vi "Config Measure Event.vi"(0 "VISA resource name":refnum<visa-resource-name>, 1 "Configure Measurement (Disable)":enum8{"DISABLE", "ENABLE", "ASYNC"}(ring), 2 "Buffer 1":string, 3 "Buffer 2":string, 5 "Node In":string, 7 "Channel (Channel A)":T1, 9 "Function (Current)":T2(ring), 11 "error in":errorcluster, 12 "Measure Input Event":string="0") -> (4 "VISA resource name out":refnum<visa-resource-name>, 6 "Node Out":string, 14 "Command String":string, 15 "error out":errorcluster)   [LabVIEW 2009, in "Keithley 2600 Series.lvlib"]
doc: "This VI configures measurements for a subsequent sweep.\n\n<b>Functions and Attributes Used</b>\nsmuX.trigger.measure.action\nsmuX.trigger.measure.i( )\nsmuX.trigger.measure.v( )\nsmuX.trigger.measure.iv( )\nsmuX.trigger.measure.p( )\nsmuX.trigger.measure.r( )"
uses:
  <instrlib>/Keithley 2600 Series/Keithley 2600 Series.lvlib
  <instrlib>/Keithley 2600 Series/Public/Channel.ctl
  <instrlib>/Keithley 2600 Series/Private/GlobalVariables.vi
panel:
  # "(c) 2008 Keithley Instruments, Inc.  ALL RIGHTS RESERVED."
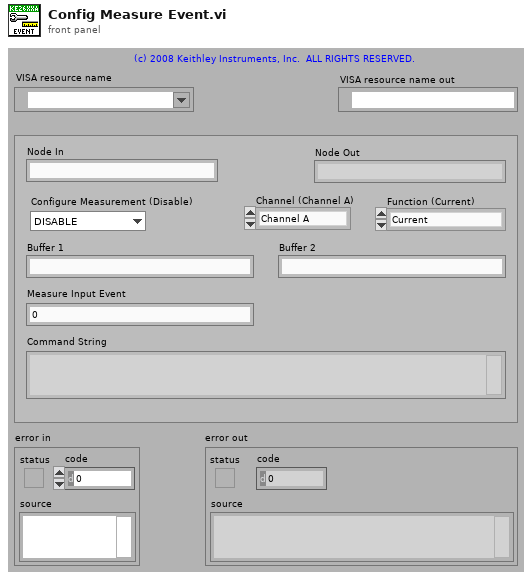
[diagram p1: front panel]
types:
  T1 = typedef "Keithley 2600 Series.lvlib/Channel.ctl" = enum32{"Channel A", "Channel B"}
  T2 = enum16{"Current", "Voltage", "IV", "Resistance", "Power"}
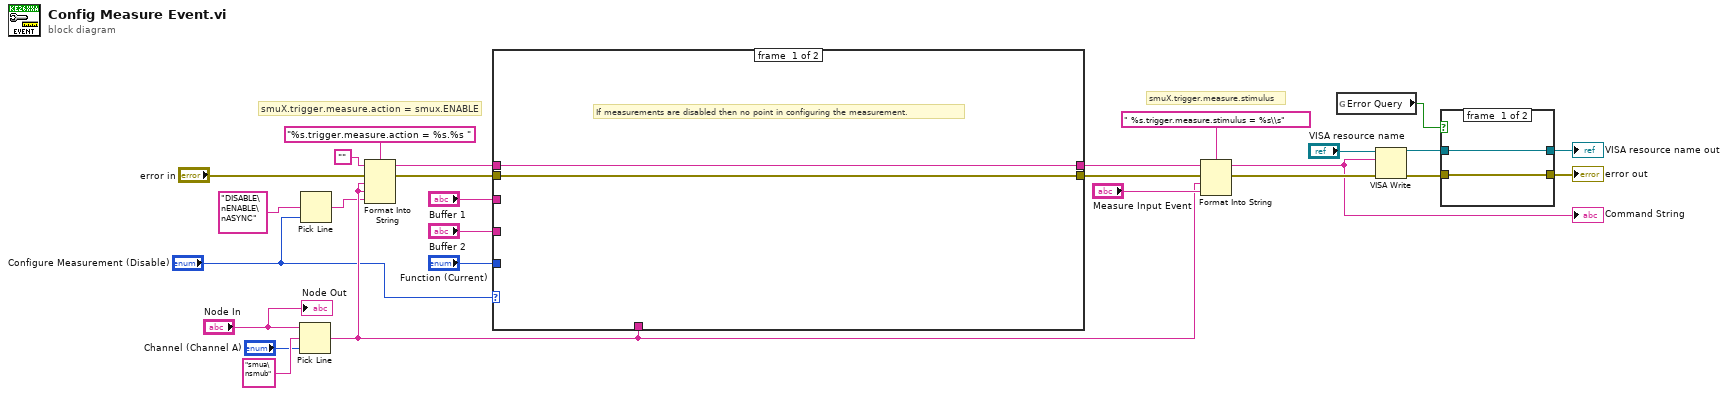
[diagram p0: block diagram]
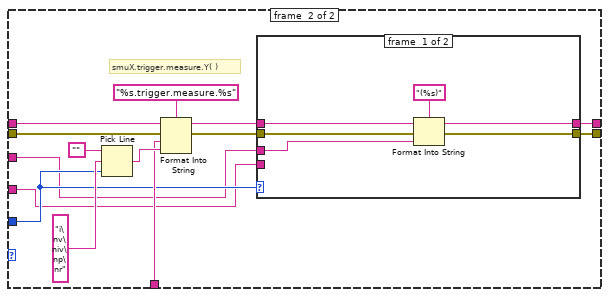
[diagram p2: hidden frame]
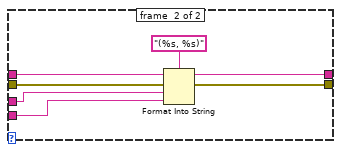
[diagram p3: hidden frame]
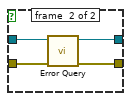
[diagram p4: hidden frame]
diagram:
  # "smuX.trigger.measure.stimulus"
  # "smuX.trigger.measure.action = smux.ENABLE"
  n1 = Pick Line(string ("")="Node In", multi-line string="smua\nsmub", line index="Channel (Channel A)") -> (output string=w10:string)
  n2 = Pick Line(multi-line string="DISABLE\nENABLE\nASYNC" ("true string"), line index="Configure Measurement (Disable)") -> (output string=w6:string)  [unwired: 1 in]
  n3 = Format Into String(format string="%s.trigger.measure.action = %s.%s ", initial string="", error in="error in", w10, w10, w6) -> (resulting string=w18:string, error out=w17:errorcluster)
  n4 = case shown="\"ENABLE\"" "Configure Measurement (Disable)" {
    tunnel: [w28 w42] -> w13
    tunnel: [w29 w41] -> w12
    tunnel: w10 -> [_ w36]
    tunnel: w18 -> [w29 w35]
    tunnel: w17 -> [w28 w34]
    tunnel: "Function (Current)" -> [_ w32]
    tunnel: "Buffer 1" -> [_ w31]
    tunnel: "Buffer 2" -> [_ w30]
    frame #0 {
      # "If measurements are disabled then no point in configuring the measurement."
    }
    frame #1 {
      # "smuX.trigger.measure.Y( )"
      n5 = Pick Line(string ("")="", multi-line string="i\nv\niv\np\nr", line index=w32) -> (output string=w39:string)
      n6 = Format Into String(format string="%s.trigger.measure.%s", initial string=w35, error in=w34, w36, w39) -> (resulting string=w37:string, error out=w38:errorcluster)
      n7 = case shown="\"Current\", \"Voltage\", \"Resistance\", \"Power\", Default" w32 {
        tunnel: w37 -> [w48 w55]
        tunnel: w38 -> [w47 w54]
        tunnel: w31 -> [w46 w53]
        tunnel: [w45 w52] -> w41
        tunnel: [w44 w51] -> w42
        tunnel: w30 -> [_ w50]
        frame #0 {
          n8 = Format Into String(format string="(%s)", initial string=w48, error in=w47, w46) -> (resulting string=w45:string, error out=w44:errorcluster)
        }
        frame #1 {
          n9 = Format Into String(format string="(%s, %s)", initial string=w55, error in=w54, w53, w50) -> (resulting string=w52:string, error out=w51:errorcluster)
        }
      }
    }
  }
  n10 = Format Into String(format string=" %s.trigger.measure.stimulus = %s\\s", initial string=w12, error in=w13, w10, "Measure Input Event") -> (resulting string=w8:string, error out=w9:errorcluster)
  "Command String" <- w8
  n11 = global read "GlobalVariables.vi" "Error Query"() -> (w24:bool)
  n12 = VISA Write(VISA resource name="VISA resource name", write buffer=w8, error in (no error)=w9) -> (VISA resource name out=w22:refnum<visa-resource-name>, error out=w23:errorcluster)  [unwired: 1 out]
  n13 = case shown="True" w24 {
    tunnel: w22 -> [w58 w62]
    tunnel: w23 -> [w57 w61]
    tunnel: [w58 w60] -> w21
    tunnel: [w57 w59] -> w20
    frame #0 {
    }
    frame #1 {
      n14 = call <instrlib>:"Error Query.vi"("error in (no error)"=w61, "VISA resource name"=w62) -> ("error out"=w59:errorcluster, "VISA resource name out"=w60:refnum<visa-resource-name>)  [unwired: 8 out]
    }
  }
  "VISA resource name out" <- w21
  "error out" <- w20
  "Node Out" <- "Node In"
